vi "FPGA Main.vi"() -> ()   [LabVIEW 2018]
uses:
  <vilib>/rvi/Emulation/niFpgaGetClockAttributes.vi
  <vilib>/rvi/Emulation/niFpgaSctlEmulationGetInTimedLoop.vi
  <vilib>/rvi/Emulation/niFpgaEmulationReportErrorSimple.vi
  <vilib>/rvi/eio/common/nirviEmuTemplateMethod_errors.vi
  <vilib>/rvi/Emulation/niFpgaCriticalErrorInLSC.vi
  <vilib>/eio/EIONode/EIONode.xnode
panel:
  out "Read Coil":i16
  in  "Voice Coil Voltage":u16(slide) scale=0.0..65565.0
  in  "Amplifier On/Off":bool
  out "Cap Probe Voltage":u16
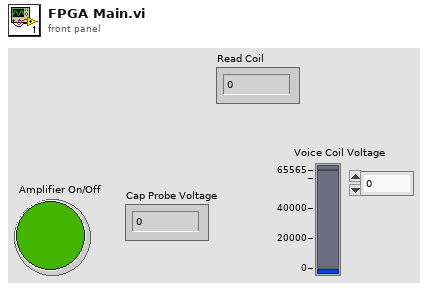
[diagram p1: front panel]
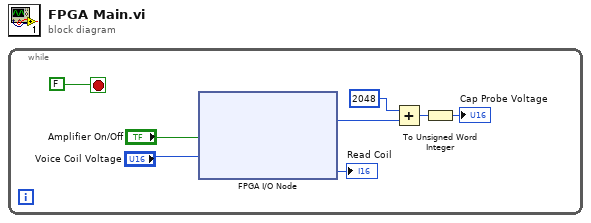
[diagram p0: block diagram]
diagram:
  n1 = while {
    stop <- FALSE stop-if-true
    n2 = xnode "FPGA I/O Node"("ConnectorA/DIO9"="Amplifier On/Off", "ConnectorA/AO1"="Voice Coil Voltage") -> ("ConnectorC/AI0"=w7:i16, "ConnectorC/AI1"=→"Read Coil":i16)  [unwired: 4 in, 4 out]
    n3 = Add(x=i16 2048, y=w7) -> (x+y=w8:i16)
    n4 = To Unsigned Word Integer(number=w8) -> (unsigned 16bit integer=→"Cap Probe Voltage":u16)
  }
